vi "CheckFoldExit_CreatFold1.vi"(0 "File in":path, 1 "FileOrFold¡H":bool) -> (2 "file or folder exists?":bool caption="文件或文件夹存在？", 3 "File out":path, 4 "Fold out":path)   [LabVIEW 2014]
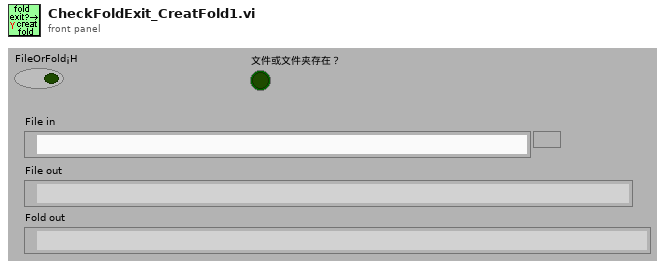
[diagram p1: front panel]
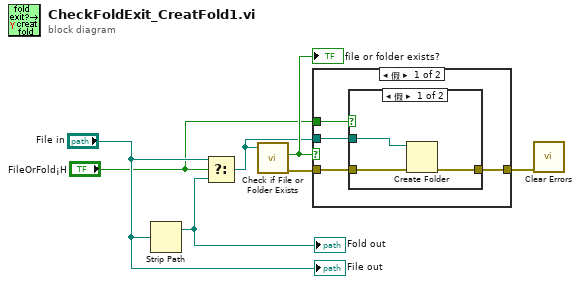
[diagram p0: block diagram]
diagram:
  n1 = Strip Path(path="File in") -> (stripped path=w3:path)  [unwired: 1 out]
  "Fold out" <- w3
  n2 = Select(t="File in", s="FileOrFold¡H", f=w3) -> (s? t:f=w6:path)
  n3 = call <vilib>:"Check if File or Folder Exists.vi"("path"=w6) -> ("error out"=w5:errorcluster, "file or folder exists?"=w7:bool)  [unwired: 1 in, 8 out]
  "file or folder exists?" <- w7
  n4 = case shown="假" w7 {
    tunnel: w6 -> [w11 _]
    tunnel: w5 -> [w10 w16]
    tunnel: [w9 w16] -> w4
    tunnel: "FileOrFold¡H" -> [w8 _]
    frame False {
      n5 = case shown="假" w8 {
        tunnel: w11 -> [w14 _]
        tunnel: w10 -> [w13 w15]
        tunnel: [w12 w15] -> w9
        frame False {
          n6 = Create Folder(path (use dialog)=w14, error in=w13) -> (error out=w12:errorcluster)  [unwired: 3 out]
        }
        frame True {
        }
      }
    }
    frame True {
    }
  }
  n7 = call <vilib>:"Clear Errors.vi"("error in (no error)"=w4) -> ()  [unwired: 5 in, 2 out]
  "File out" <- "File in"
